vi "getConnectionPoint.vi"(0 "reference":refnum<class "PointNode.lvclass">, 1 "direction":refnum<class "Direction.lvclass">, 5 "error in (no error)":errorcluster) -> (14 "reference out":refnum<class "PointNode.lvclass">, 15 "point2D":T1 {"y" format="%.2f"; "x" format="%.2f"}, 19 "error out":errorcluster)   [LabVIEW 2014, in "PointNode.lvclass"]
doc: "public Point2D getConnectionPoint(Direction d)"
uses:
  <resource>/Framework/Providers/Open_GDS/UML/PointNode_class/PointNode.lvclass
  <resource>/Framework/Providers/Open_GDS/UML/Direction_class/Direction.lvclass
  <resource>/Framework/Providers/Open_GDS/UML/General/Point/Point Point2D.ctl
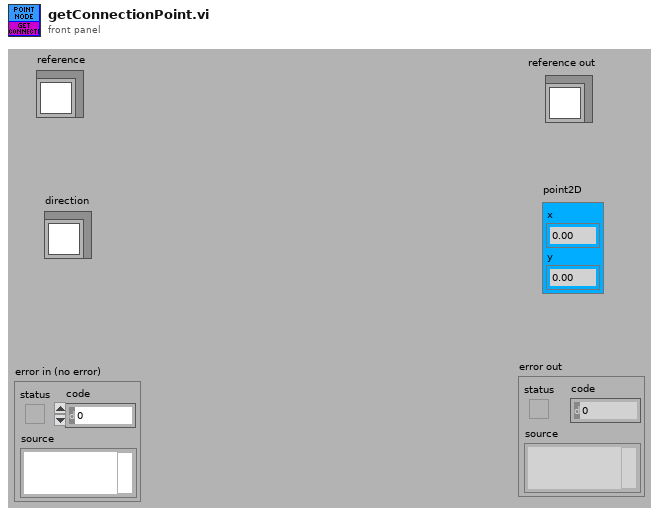
[diagram p1: front panel]
types:
  T1 = typedef "Point Point2D.ctl" = cluster{"x":dbl, "y":dbl}
  T2 = typedef "PointNode.lvclass/ObjectAttributes.ctl" = cluster{"point":T1}
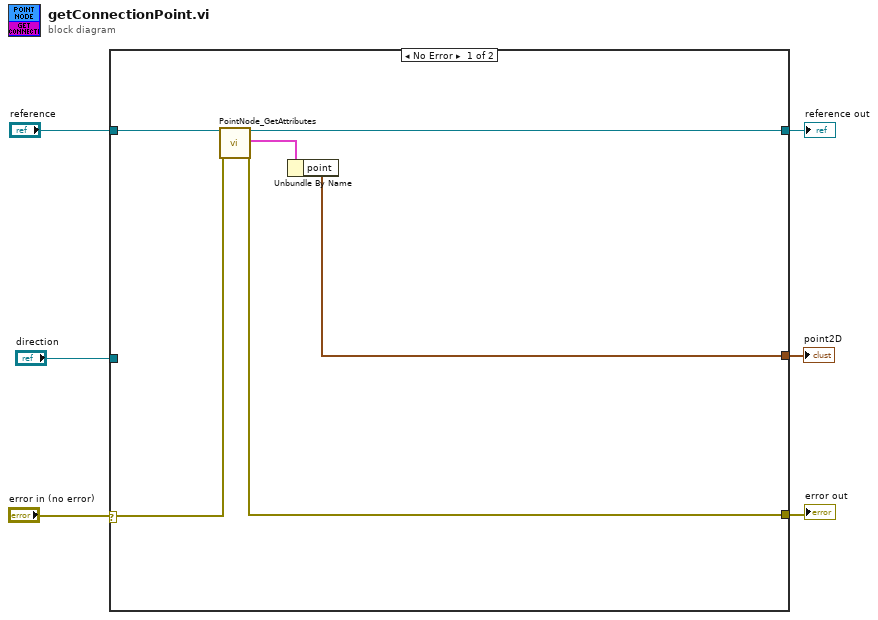
[diagram p0: block diagram]
diagram:
  n1 = case shown="No Error" "error in (no error)" {
    selector: "error in (no error)" -> [w8 w13]
    tunnel: "reference" -> [w12 w14]
    tunnel: [w11 w13] -> w5
    tunnel: [w10 w14] -> w4
    tunnel: [w9 _] -> w2
    tunnel: "direction" -> [_ _]
    frame No Error {
      n2 = call <resource>:"PointNode_GetAttributes.vi"("reference in"=w12, "error in (no error)"=w8) -> ("reference out"=w10:refnum<class "PointNode.lvclass">, "Data"=w7:T2, "error out"=w11:errorcluster)  [unwired: 1 in, 14 out]
      n3 = Unbundle By Name(w7) -> ("point"=w9:T1)
    }
    frame Error {
    }
  }
  "reference out" <- w4
  "error out" <- w5
  "point2D" <- w2
